vi "STM_Client.vi"(8 "error in (no error)":errorcluster, 9 "data to send":string, 10 "Command":T1, 11 "address":string) -> (0 "error out":errorcluster, 1 "data received from server":string)   [LabVIEW 2016, in "LockinRemoteControl.lvclass"]
uses:
  LockinRemoteControl.lvclass
  Typedefs/Remote-SMO-Commands-Enum.ctl
  <vilib>/NI/STM/TCP/TCP Read Options.ctl
  <vilib>/NI/STM/TCP/Read Meta Data (TCP Ref).vi
  <vilib>/NI/STM/TCP/Get Connection Reference (TCP).vi
  <vilib>/NI/STM/TCP/Read Meta Data (TCP Clst).vi
  <vilib>/NI/STM/TCP/Write Message (TCP).vi
  <vilib>/NI/STM/TCP/Read Message (TCP).vi
  <userlib>/_OpenG.lib/error/error.llb/Filter Error Codes (Array)__ogtk.vi
  <vilib>/NI/STM/NI STM.lvlib
panel:
  out "Numeric 2":i32
  out "Numeric":i32
  out "since last call ms":u32
  out "duration ms":u32
  out "available commands = enum?":bool
  out "meta data (available commands)":string[](array[string])
  # "CLIENT (API)"
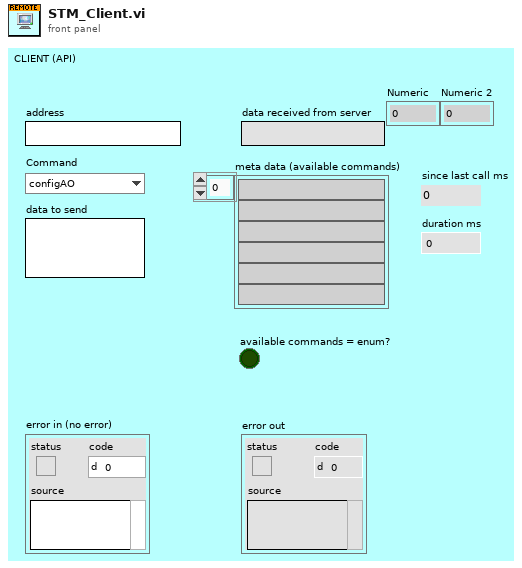
[diagram p1: front panel]
types:
  T1 = typedef "LockinRemoteControl.lvclass/Remote-SMO-Commands-Enum.ctl" = enum16{"configAO", "configREF", "configREFfilter", "configIVmode", "configRemote", "configReset", "configSampling", "assertTrigger", "getAO", "getAI", "getResults", "getTrigger", "getIVmode", "getSampling", "getAOconfig", "getREFconfig", "getREFfilter", "ACK", "UNK", "CLOSE", "configGain", "getGain"}
  T2 = typedef "NI STM.lvlib/TCP Read Options.ctl" = cluster{"ignore timeout error":bool, "timeout ms (1000)":i32}
  T3 = typedef "NI STM.lvlib/MetaDataElement.ctl" = string
  T4 = typedef "NI STM.lvlib/TCP Connection Info.ctl" = cluster{"connection ID":refnum<k5>, "meta data":T3[]}
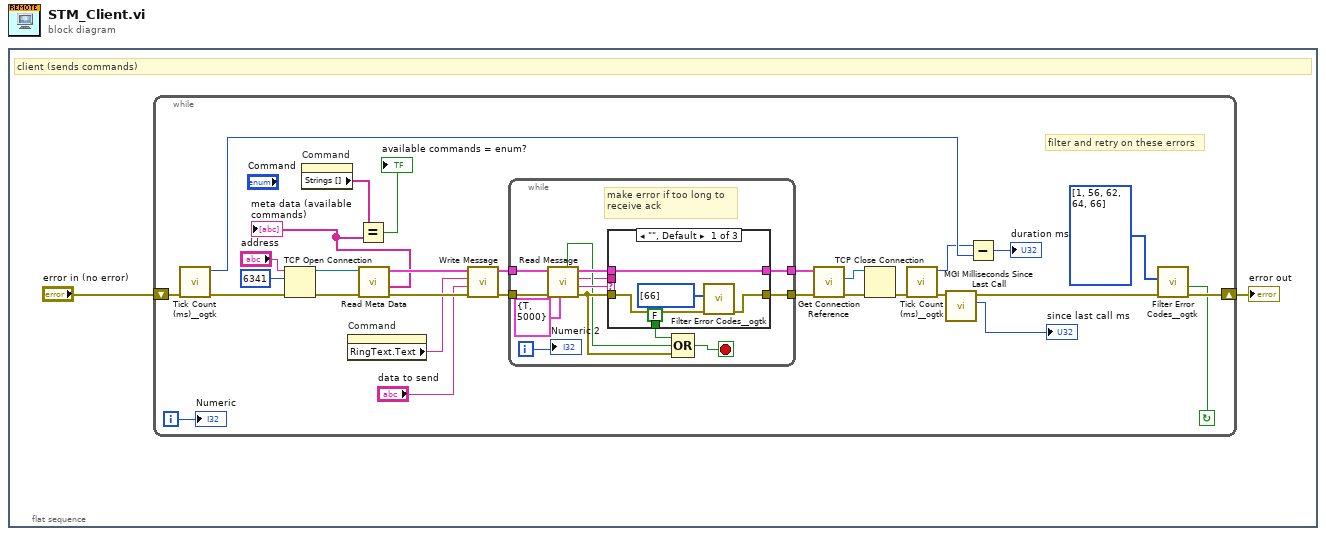
[diagram p0: block diagram]
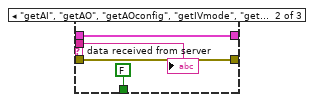
[diagram p2: hidden frame]
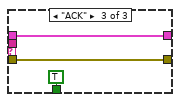
[diagram p3: hidden frame]
diagram:
  n1 = flat-sequence {
    frame #0 {
      # "client (sends commands)"
      n2 = while {
        shift-right: [w7] -> w1
        shift-left: "error in (no error)" -> [w15]
        i -> [w3]
        stop <- w6 continue-if-true
        # "filter and retry on these errors"
        n3 = call <userlib>:"Tick Count (ms)__ogtk.vi"("error in (no error)"=w15) -> ("error out"=w20:errorcluster, "millisecond timer value"=w13:u32)  [unwired: 9 in]
        n4 = TCP Open Connection(address="address", remote port or service name=u16 6341, error in (no error)=w20) -> (connection ID=w27:refnum<k5>, error out=w28:errorcluster)  [unwired: 2 in]
        n5 = property on="Command" class="Enum (strict)"() -> ("Strings []"=w26:string[])  [unwired: 2 in, 2 out]
        n6 = property on="Command" class="Enum (strict)"() -> ("RingText.Text"=w19:string)  [unwired: 2 in, 2 out]
        n7 = call-poly <vilib>:"Read Meta Data.vi"("error in"=w28, "connection ID"=w27) -> ("error out"=w31:errorcluster, "meta data"=w23:T3[], "connection info out"=w32:T4)  [unwired: 7 in]
        "meta data (available commands)" <- w23
        n8 = Equal?(x=w26, y=w23) -> (x = y?=→"available commands = enum?":bool)
        n9 = call-poly <vilib>:"Write Message.vi"("error in"=w31, "data"="data to send", "name"=w19, "connection info in"=w32) -> ("error out"=w30:errorcluster, "connection info out"=w29:T4)  [unwired: 6 in]
        n10 = while {
          tunnel: w30 -> [w45]
          tunnel: w29 -> [w44]
          tunnel: [w42] -> w11
          tunnel: [w40] -> w10
          i -> [w33]
          stop <- w39 stop-if-true
          # "make error if too long to\nreceive ack"
          n11 = call-poly <vilib>:"Read Message.vi"("options"=T2 {"ignore timeout error"=TRUE, "timeout ms (1000)"=5000}, "error in"=w45, "connection info in"=w44) -> ("error out"=w38:errorcluster, "name"=w43:T3, "data string"=w36:string, "connection info out"=w41:T4, "timed out?"=w37:bool)  [unwired: 1 in, 3 out]
          n12 = case shown="\"\", Default" w43 {
            tunnel: w38 -> [w47 w54 w56]
            tunnel: [w49 w54 w56] -> w42
            tunnel: w41 -> [w50 w53 w57]
            tunnel: [w50 w53 w57] -> w40
            tunnel: w36 -> [_ w52 _]
            tunnel: [FALSE ("value") FALSE ("value") TRUE ("value")] -> w34
            frame "", Default {
              n13 = call-poly <userlib>:"Filter Error Codes__ogtk.vi"("Error In"=w47, "Error Codes to Filter"=i32[] [66]) -> ("Error Out"=w49:errorcluster)  [unwired: 7 in, 2 out]
            }
            frame "getAI", "getAO", "getAOconfig", "getIVmode", "getREFconfig", "getREFfilter", "getResults", "getSampling", "getTrigger" {
              "data received from server" <- w52
            }
            frame "ACK" {
            }
          }
          n14 = Compound Arithmetic op=OR(w34, w37, w38) -> (w39:bool)
          "Numeric 2" <- w33
        }
        n15 = call-poly <vilib>:"Get Connection Reference.vi"("error in"=w11, "connection info in"=w10) -> ("error out"=w21:errorcluster, "connection ID out"=w9:refnum<k5>)  [unwired: 7 in, 1 out]
        n16 = TCP Close Connection(connection ID=w9, error in (no error)=w21) -> (error out=w18:errorcluster)  [unwired: 1 in, 1 out]
        n17 = call <userlib>:"Tick Count (ms)__ogtk.vi"("error in (no error)"=w18) -> ("error out"=w16:errorcluster, "millisecond timer value"=w12:u32)  [unwired: 9 in]
        n18 = call <userlib>:"MGI Milliseconds Since Last Call.vi"("Error In"=w16) -> ("ms"=→"since last call ms":u32, "Error Out"=w8:errorcluster)  [unwired: 5 in]
        n19 = Subtract(x=w12, y=w13) -> (x-y=→"duration ms":u32)
        n20 = call-poly <userlib>:"Filter Error Codes__ogtk.vi"("Error In"=w8, "Error Codes to Filter"=i32[] [1, 56, 62, 64, 66]) -> ("Error Out"=w7:errorcluster, "Error Filtered?"=w6:bool)  [unwired: 7 in, 1 out]
        "Numeric" <- w3
      }
      "error out" <- w1
    }
  }
